vi "Test Array.vi"() -> ()   [LabVIEW 2010]
uses:
  <vilib>/MDSplus/Library/Data/Array/Int8Array/Int8Array Create.vi
  <vilib>/MDSplus/Library/MDSplus.lvlib
panel:
  out "I8 array out":i8[](array[numeric])
  in  "I8 array in":i8[](array[numeric])
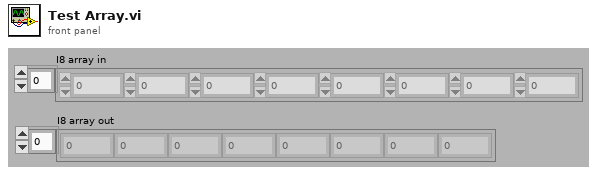
[diagram p1: front panel]
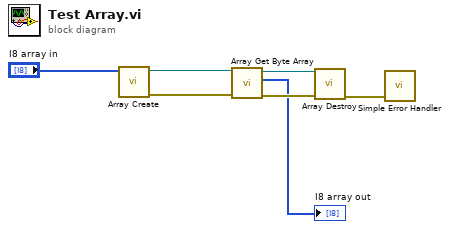
[diagram p0: block diagram]
diagram:
  n1 = call-poly <vilib>:"Array Create.vi"("I8 array in"="I8 array in") -> ("error out"=w5:errorcluster, "Int8Array DVR out"=w6:refnum<data-value>)  [unwired: 9 in]
  n2 = call <vilib>:"Array Get Byte Array.vi"("error in (no error)"=w5, "Array DVR in"=w6) -> ("error out"=w3:errorcluster, "I8 array out"=→"I8 array out":i8[], "Array DVR out"=w4:refnum<data-value>)  [unwired: 6 in, 1 out]
  n3 = call <vilib>:"Array Destroy.vi"("error in (no error)"=w3, "Array DVR in"=w4) -> ("error out"=w1:errorcluster)  [unwired: 9 in]
  n4 = call <vilib>:"Simple Error Handler.vi"("error in (no error)"=w1) -> ()  [unwired: 4 in, 5 out]
